vi "Voltage - On Demand Output.vi"() -> ()   [LabVIEW 2012]
doc: "This example demonstrates how to generate a user-defined voltage using the analog output of a DAQ device."
uses:
  <vilib>/DAQmx/write.llb/DAQmx Write (Analog 1D DBL NChan 1Samp).vi
  <vilib>/DAQmx/create/channels.llb/DAQmx Create Channel (AO-Voltage-Basic).vi
  <vilib>/DAQmx/miscellaneous.llb/DAQmx Fill In Error Info.vi
panel:
  in  "Output Array":dbl[](array[numeric])=[1.0, 3.0]
  in  "Stop":bool
  in  "Max Voltage":dbl=5.0
  in  "Min Voltage":dbl
  in  "Physical Channel(s)":tag="Dev5/ao0:1"
  # "Channel Settings"
  # "Output"
  # "The number of elements in the output array\nmust equal the number of channels in the task."
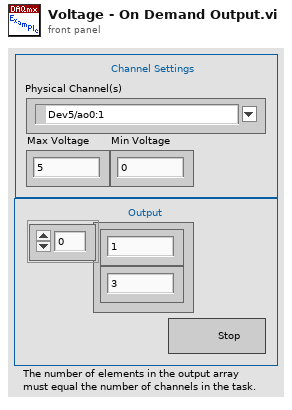
[diagram p1: front panel]
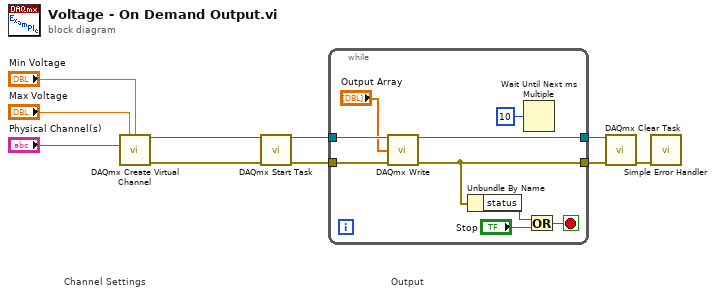
[diagram p0: block diagram]
diagram:
  # "Output"
  # "Channel Settings"
  n1 = call-poly <vilib>:"DAQmx Create Virtual Channel.vi"("maximum value"="Max Voltage", "minimum value"="Min Voltage", "physical channels"="Physical Channel(s)") -> ("task out"=w6:refnum<k21>, "error out"=w5:errorcluster)  [unwired: 11 in]
  n2 = call <vilib>:"DAQmx Start Task.vi"("task/channels in"=w6, "error in"=w5) -> ("task out"=w4:refnum<k21>, "error out"=w3:errorcluster)  [unwired: 12 in]
  n3 = while {
    tunnel: w4 -> [w19]
    tunnel: w3 -> [w18]
    tunnel: [w13] -> w2
    tunnel: [w17] -> w1
    stop <- w12 stop-if-true
    n4 = call-poly <vilib>:"DAQmx Write.vi"("task/channels in"=w19, "data"="Output Array", "error in"=w18) -> ("task out"=w17:refnum<k21>, "error out"=w13:errorcluster)  [unwired: 10 in, 1 out]
    n5 = Unbundle By Name(w13) -> ("status"=w15:bool)
    n6 = Wait Until Next ms Multiple(millisecond multiple=u32 10) -> ()  [unwired: 1 out]
    n7 = Or(x=w15, y="Stop") -> (x .or. y?=w12:bool)
  }
  n8 = call <vilib>:"DAQmx Clear Task.vi"("task in"=w1, "error in"=w2) -> ("error out"=w10:errorcluster)  [unwired: 13 in]
  n9 = call <vilib>:"Simple Error Handler.vi"("error in (no error)"=w10) -> ()  [unwired: 4 in, 5 out]
